vi "aft_Get_Memory_Ref.vi"(10 "memory name":string, 11 "target ref":refnum<vi>) -> (1 "exist?":bool, 2 "memory name out":string, 3 "memory ref":refnum<vi>)   [LabVIEW 2017, in "NI_AdaptiveFilter.lvlib"]
uses:
  <vilib>/addons/Adaptive Filters/NI_AdaptiveFilter.lvlib
  <vilib>/rvi/ClientSDK/Core/Script/Memory/ProjectItem/Private/nirviPiMemory_CommitGlobal.vi
  <vilib>/rvi/ClientSDK/Core/Script/Memory/ProjectItem/Private/nirviPiMemory_OpenWithName2.vi
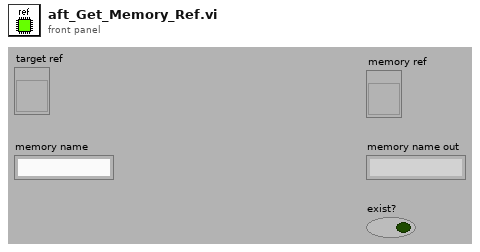
[diagram p1: front panel]
types:
  T1 = typedef "nirviPiMemory_State.ctl" = cluster{"Item":refnum<vi>, "Memory Block":T2, "Dirty":bool, "XNode":refnum<vi>, "Init Data String":string}
  T2 = typedef "niFpgaContainerState.ctl" = cluster{"displayName":string, "hardwareName":string, "dataType":T3, "elementTypeDescriptor":variant, "terminalTypeDescriptor":variant, "requestedNumberOfElements":u32, "memoryType":T4, "arbitrationForInterfaceA":T5, "numberOfElementsPerRead":u32, "arbitrationForInterfaceB":T5, "numberOfElementsPerWrite":u32, "VI_Defined":bool, "type":T6, "initializationParameters":T7, "disableOnOverflow/Underflow":bool, "interfaceConfiguration":T8, "controlLogic":T9, "actualNumberOfElements":u32, "dramSelection":string, "dramMaxOustandingRequests":i32, "dramIncludeByteEnables":bool, "dramGrantTime":u32, "fullEmulation":bool, "memoryInMultipleClockDomains":bool, "memoryLatency":T10}
  T3 = typedef "niFpgaDataTypeControl.ctl" = enum32{"Boolean", "I8", "I16", "I32", "I64", "U8", "U16", "U32", "U64", "FXP", "CustomControl", "SGL"}
  T4 = typedef "niFpgaContainerImplementationControl.ctl" = enum16{"Flip-Flops", "Look-Up Table", "Block Memory", "DRAM"}
  T5 = typedef "niFpgaContainerArbitrationOptionsControl.ctl" = enum16{"Always Arbitrate", "Arbitrate if Multiple Requestors Only", "Never Arbitrate"}
  T6 = typedef "niFpgaTransferTypeControl.ctl" = enum16{"Target-Scoped", "Host to Target - DMA", "Target to Host - DMA", "Peer to Peer Reader", "Peer to Peer Writer", "Bidirectional"}
  T7 = typedef "niFpgaContainerInitializationParameters.ctl" = cluster{"initialized":bool, "VI_Path":path, "initialData":variant}
  T8 = typedef "niFpgaMemoryInterfaceConfiguration.ctl" = enum16{"Read A-Write B", "Read A-Read B"}
  T9 = typedef "niFpgaFifoControlLogicControl.ctl" = enum16{"Slice Fabric", "Target Optimal", "Built-in"}
  T10 = typedef "niFpgaContainerMemoryLatencyControl.ctl" = u16
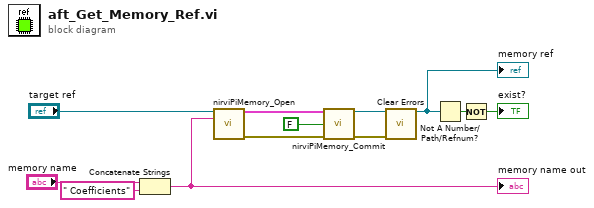
[diagram p0: block diagram]
diagram:
  n1 = Concatenate Strings("memory name", " Coefficients" ("string")) -> (w1:string)
  "memory name out" <- w1
  n2 = call-poly <vilib>:"nirviPiMemory_Open.vi"("Parent Item"="target ref", "Memory Name"=w1) -> ("Memory Reference"=w6:T1, "error out"=w8:errorcluster)  [unwired: 12 in]
  n3 = call-poly <vilib>:"nirviPiMemory_Commit.vi"("Reference"=w6, "Close Reference?"=FALSE, "error in (no error)"=w8) -> ("ProjectItem"=w7:refnum<vi>, "error out"=w4:errorcluster)  [unwired: 11 in]
  "memory ref" <- w7
  n4 = call <vilib>:"Clear Errors.vi"("error in (no error)"=w4) -> ()  [unwired: 5 in, 2 out]
  n5 = Not A Number/Path/Refnum?(number/path/refnum=w7) -> (NaN/Path/Refnum?=w11:bool)
  n6 = Not(x=w11) -> (.not. x?=→"exist?":bool)
